vi "Example.vi"() -> ()   [LabVIEW 2019, in "MicronManager.lvclass"]
uses:
  MicronManager.lvclass
panel:
  out "Responses":string[](array[string])
  out "Services":string[](array[string])
  in  "Service List":path
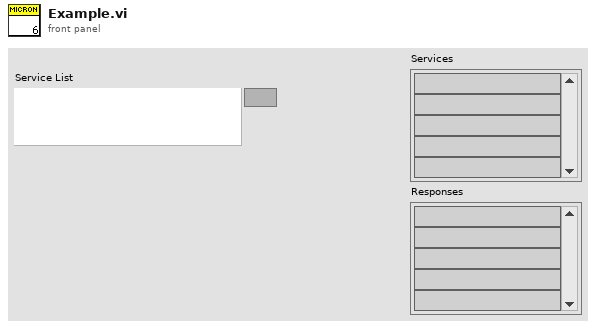
[diagram p1: front panel]
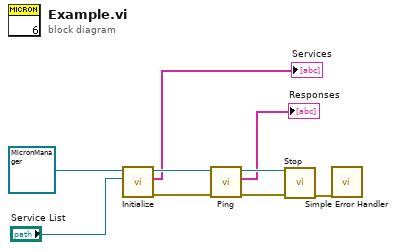
[diagram p0: block diagram]
diagram:
  n1 = call-dynamic "Initialize.vi"("Service List"="Service List", "MicronManager in"=refnum<class "MicronManager.lvclass"> refnum) -> ("error out"=w9:errorcluster, "Services"=→"Services":string[], "MicronManager out"=w7:refnum<class "MicronManager.lvclass">)  [unwired: 7 in]
  n2 = call-dynamic "Ping.vi"("error in (no error)"=w9, "MicronManager in"=w7) -> ("error out"=w8:errorcluster, "Responses"=→"Responses":string[], "MicronManager out"=w6:refnum<class "MicronManager.lvclass">)  [unwired: 7 in]
  n3 = call-dynamic "Stop.vi"("error in (no error)"=w8, "MicronManager in"=w6) -> ("error out"=w1:errorcluster)  [unwired: 8 in, 1 out]
  n4 = call <vilib>:"Simple Error Handler.vi"("error in (no error)"=w1) -> ()  [unwired: 4 in, 5 out]
